vi "RP proccess data.vi"() -> ()   [LabVIEW 2015]
uses:
  <vilib>/Analysis/NI_AALPro.lvlib
panel:
  in  "Integrate Bdot":bool=TRUE
  in  "Fix time delay":bool=TRUE
  in  "Time constant":dbl=0.0001 format="%#_6p"
  out "XY Graph":cluster{dbl[], "Y":dbl[]}[](graph)
  out "Error Out":errorcluster
  in  "Bdot calibration":dbl=2506.0
  in  "offset length":i32=990000
  out "Waveform Graph":waveform(dbl)[](graph)
  in  "Bdot channel":string
  in  "Signal channel":string
  in  "Bdot file":path
  in  "Signal file":path
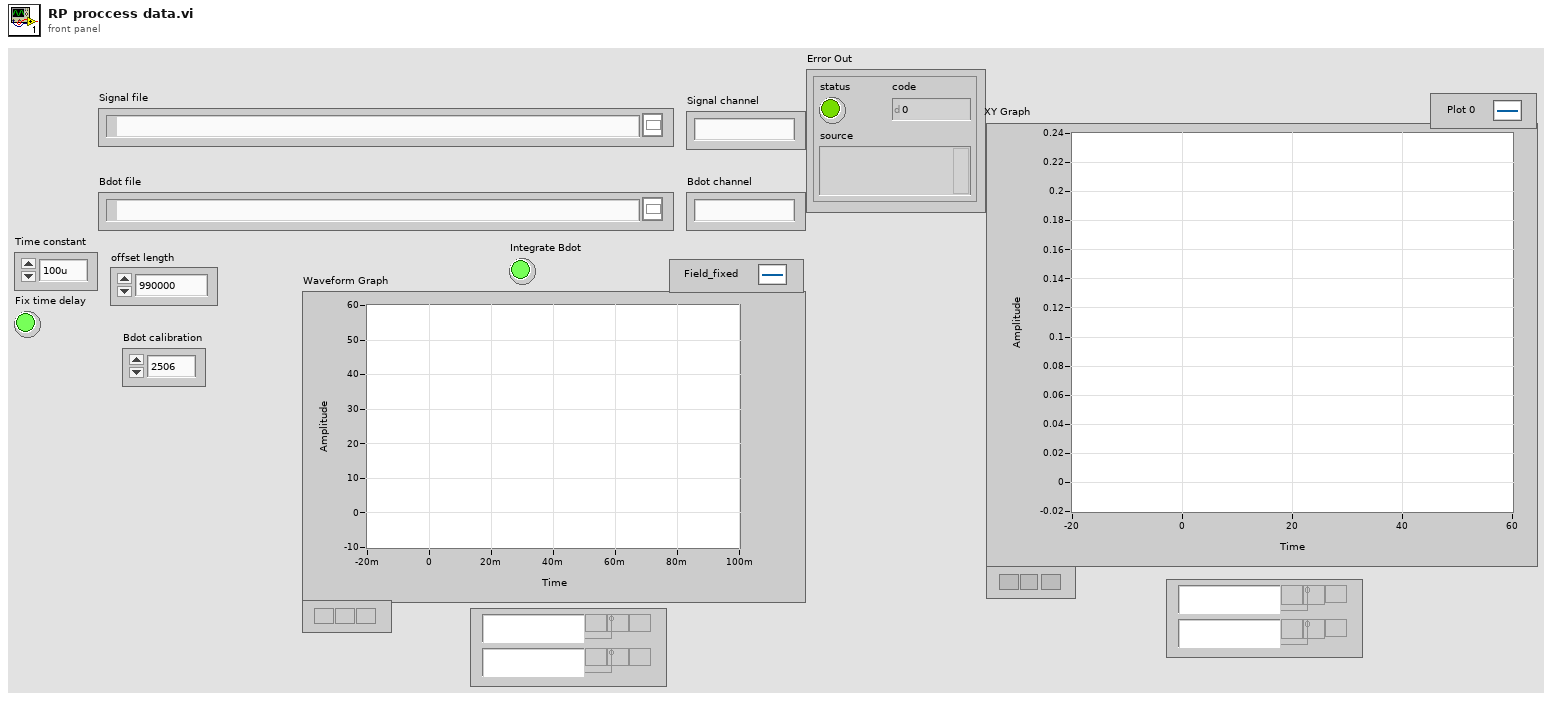
[diagram p1: front panel]
types:
  T1 = enum16{"open", "open or create", "create or replace", "create", "open (read-only)"}
  T2 = cluster{"Waveform":waveform(dbl), "Waveform":waveform(dbl)}
  T3 = cluster{"Waveform":waveform(dbl), "Waveform":waveform(dbl)}[]
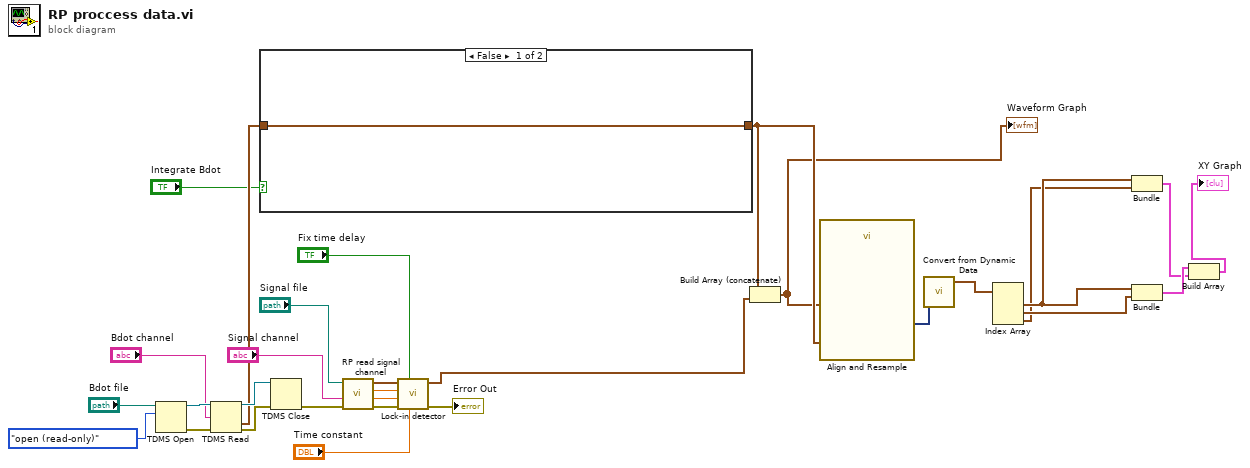
[diagram p0: block diagram]
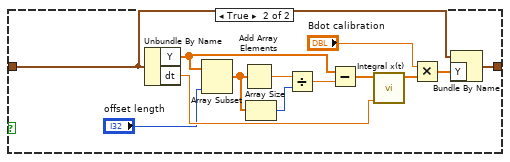
[diagram p2: hidden frame]
diagram:
  n1 = TDMS Open(10:T1."open (read-only)" ("operation (0:open)"), 11:"Bdot file") -> (0:w28:errorcluster, 3:w27:refnum<k34>)  [unwired: 5 in]
  n2 = TDMS Read(0:w27, 7:"Bdot channel", 11:w28) -> (4:w24:refnum<k34>, 10:w23:waveform(dbl), 15:w25:errorcluster)  [unwired: 5 in, 3 out]
  n3 = case shown="False" "Integrate Bdot" {
    tunnel: w23 -> [w31 w34]
    tunnel: [w31 w32] -> w10
    frame False {
    }
    frame True {
      n4 = Unbundle By Name(w34) -> ("Y"=w37:dbl[], "dt"=w44:dbl)
      n5 = Array Subset(array=w37, length="offset length") -> (w41:dbl[])  [unwired: 1 in]
      n6 = Add Array Elements(numeric array=w41) -> (sum=w40:dbl)
      n7 = Array Size(array=w41) -> (size(s)=w39:i32)
      n8 = Divide(x=w40, y=w39) -> (x/y=w36:dbl)
      n9 = Subtract(x=w37, y=w36) -> (x-y=w38:dbl[])
      n10 = call <vilib>:"Integral x(t).vi"("dt"=w44, "X"=w38) -> ("Integral X"=w43:dbl[])  [unwired: 8 in, 1 out]
      n11 = Multiply(x="Bdot calibration", y=w43) -> (x*y=w33:dbl[])
      n12 = Bundle By Name(cluster=w34, "Y"=w33) -> (w32:waveform(dbl))
    }
  }
  n13 = TDMS Close(8:w25, 11:w24) -> (0:w20:errorcluster)  [unwired: 1 out]
  n14 = call "RP read signal channel.vi"("Error In"=w20, "Channel name"="Signal channel", "File Path Control"="Signal file") -> ("Error Out"=w16:errorcluster, "Phase"=w17:dbl, "Frequency"=w18:dbl, "Data out"=w19:waveform(dbl))  [unwired: 3 in, 2 out]
  n15 = call "Lock-in detector.vi"("Time constant"="Time constant", "Fix time delay"="Fix time delay", "Error In"=w16, "Phase"=w17, "Frequency"=w18, "Data in"=w19) -> ("Error Out"=→"Error Out":errorcluster, "Data out"=w11:waveform(dbl)[])  [unwired: 4 in]
  n16 = Build Array (concatenate)(w10, w11) -> (w1:waveform(dbl)[])
  "Waveform Graph" <- w1
  n17 = call "Align and Resample"("Reference Signal"=w10, "Signals"=w1) -> ("Resampled Signals"=w9:dynamicdata)  [unwired: 7 in, 2 out]
  n18 = call "Convert from Dynamic Data"("Dynamic Data Type"=w9) -> ("Array of Waveform"=w8:waveform(dbl)[])  [unwired: 3 in]
  n19 = Index Array(array=w8) -> (element #1=w6:waveform(dbl), element #2=w7:waveform(dbl), element #3=w4:waveform(dbl))  [unwired: 3 in]
  n20 = Bundle("Waveform"=w6, "Waveform"=w4) -> (w3:T2)  [unwired: 1 in]
  n21 = Bundle("Waveform"=w6, "Waveform"=w7) -> (w5:T2)  [unwired: 1 in]
  n22 = Build Array(w5, w3) -> (→"XY Graph":T3)
